vi "Wavform data.vi"(8 "错误输入":errorcluster, 11 "VISA资源名称":refnum<visa-resource-name>) -> (0 "错误输出":errorcluster, 1 "数组":u8[](array[numeric]), 2 "波形图":u8[](graph), 3 "VISA资源名称输出":refnum<visa-resource-name>)   [LabVIEW 2020]
panel:
  out "返回数 2":u32
  out "长度":i32
  out "Data":string
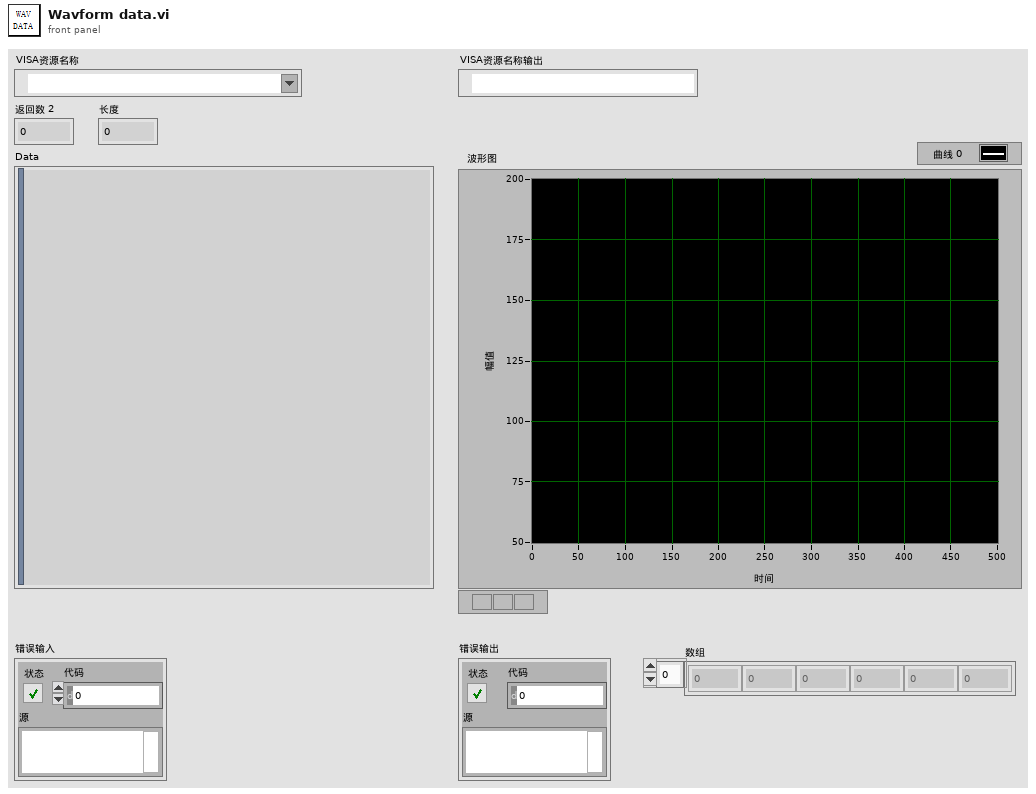
[diagram p1: front panel]
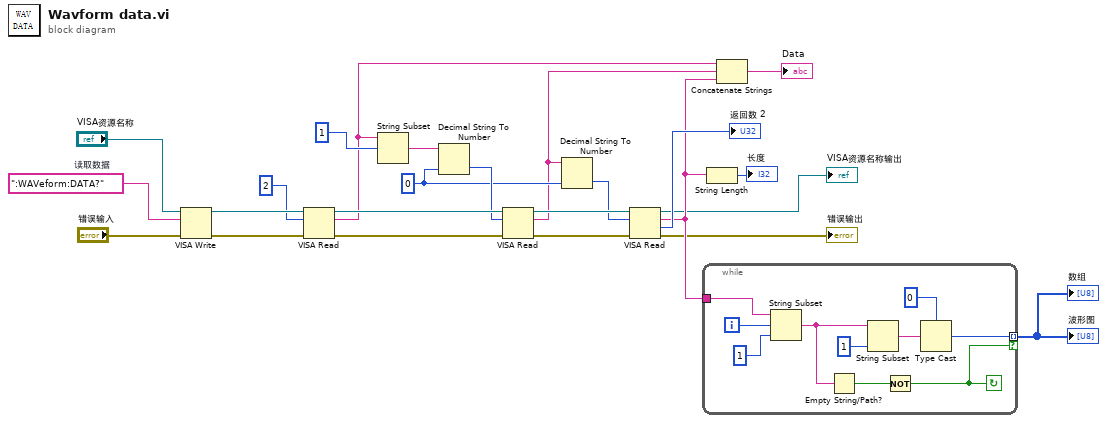
[diagram p0: block diagram]
diagram:
  w15 = u32 0 ("字节总数")
  w24 = ":WAVeform:DATA?"  # 读取数据
  n1 = VISA Write(VISA resource name="VISA资源名称", write buffer=w24, error in (no error)="错误输入") -> (VISA resource name out=w23:refnum<visa-resource-name>, error out=w22:errorcluster)  [unwired: 1 out]
  n2 = VISA Read(VISA resource name=w23, byte count=u32 2 ("字节总数"), error in (no error)=w22) -> (VISA resource name out=w18:refnum<visa-resource-name>, read buffer=w9:string, error out=w16:errorcluster)  [unwired: 1 out]
  n3 = String Subset(string=w9, offset (0)=1 ("偏移量(0)")) -> (substring=w19:string)  [unwired: 1 in]
  n4 = Decimal String To Number(string=w19, default (0L)=w15) -> (number=w17:u32)  [unwired: 1 in, 1 out]
  n5 = VISA Read(VISA resource name=w18, byte count=w17, error in (no error)=w16) -> (VISA resource name out=w14:refnum<visa-resource-name>, read buffer=w8:string, error out=w12:errorcluster)  [unwired: 1 out]
  n6 = Decimal String To Number(string=w8, default (0L)=w15) -> (number=w13:u32)  [unwired: 1 in, 1 out]
  n7 = VISA Read(VISA resource name=w14, byte count=w13, error in (no error)=w12) -> (VISA resource name out=→"VISA资源名称输出":refnum<visa-resource-name>, read buffer=w7:string, return count=→"返回数 2":u32, error out=→"错误输出":errorcluster)
  n8 = while {
    tunnel: w7 -> [w34]
    tunnel: [w28] -> w5 mode=indexing if=w25
    i -> [w32]
    stop <- w25 continue-if-true
    n9 = String Subset(string=w34, offset (0)=w32, length (rest)=1 ("长度（剩余）")) -> (substring=w29:string)
    n10 = Empty String/Path?(string/path=w29) -> (empty?=w26:bool)
    n11 = String Subset(string=w29, length (rest)=1 ("长度（剩余）")) -> (substring=w31:string)  [unwired: 1 in]
    n12 = Not(x=w26) -> (.not. x?=w25:bool)
    n13 = Type Cast(type=u8 0, x=w31) -> (*(type *) &x=w28:u8)
  }
  "波形图" <- w5
  "数组" <- w5
  n14 = String Length(string=w7) -> (length=→"长度":i32)
  n15 = Concatenate Strings(w9, w8, w7) -> (→"Data":string)
